vi "DataProcess_ChangeCatchName.vi"() -> ()   [LabVIEW 2016]
panel:
  in  "path 2":path
  out "Array 2":bool[](array[boolean])
  out "Array":string[](array[string])
  out "filenames":string[](array[string])
  in  "path":path
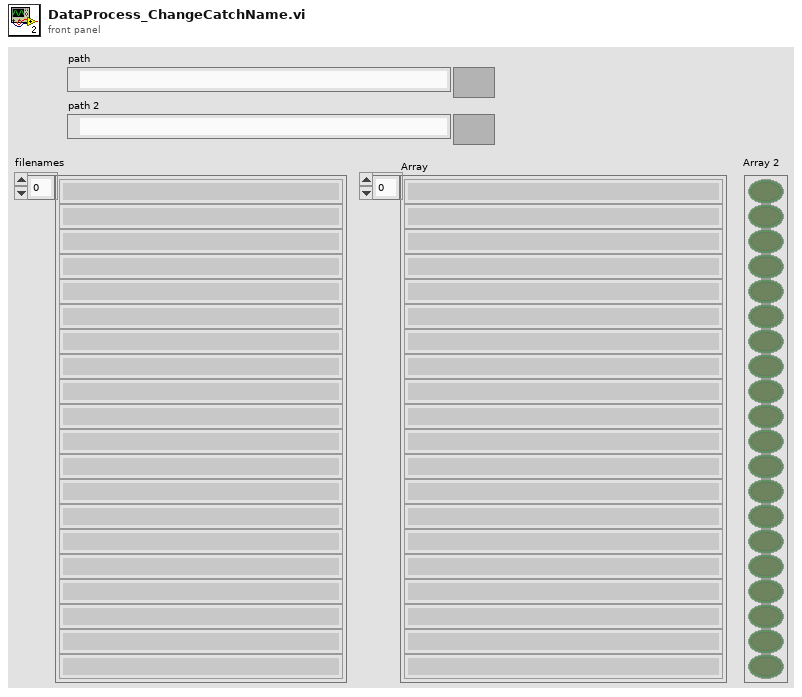
[diagram p1: front panel]
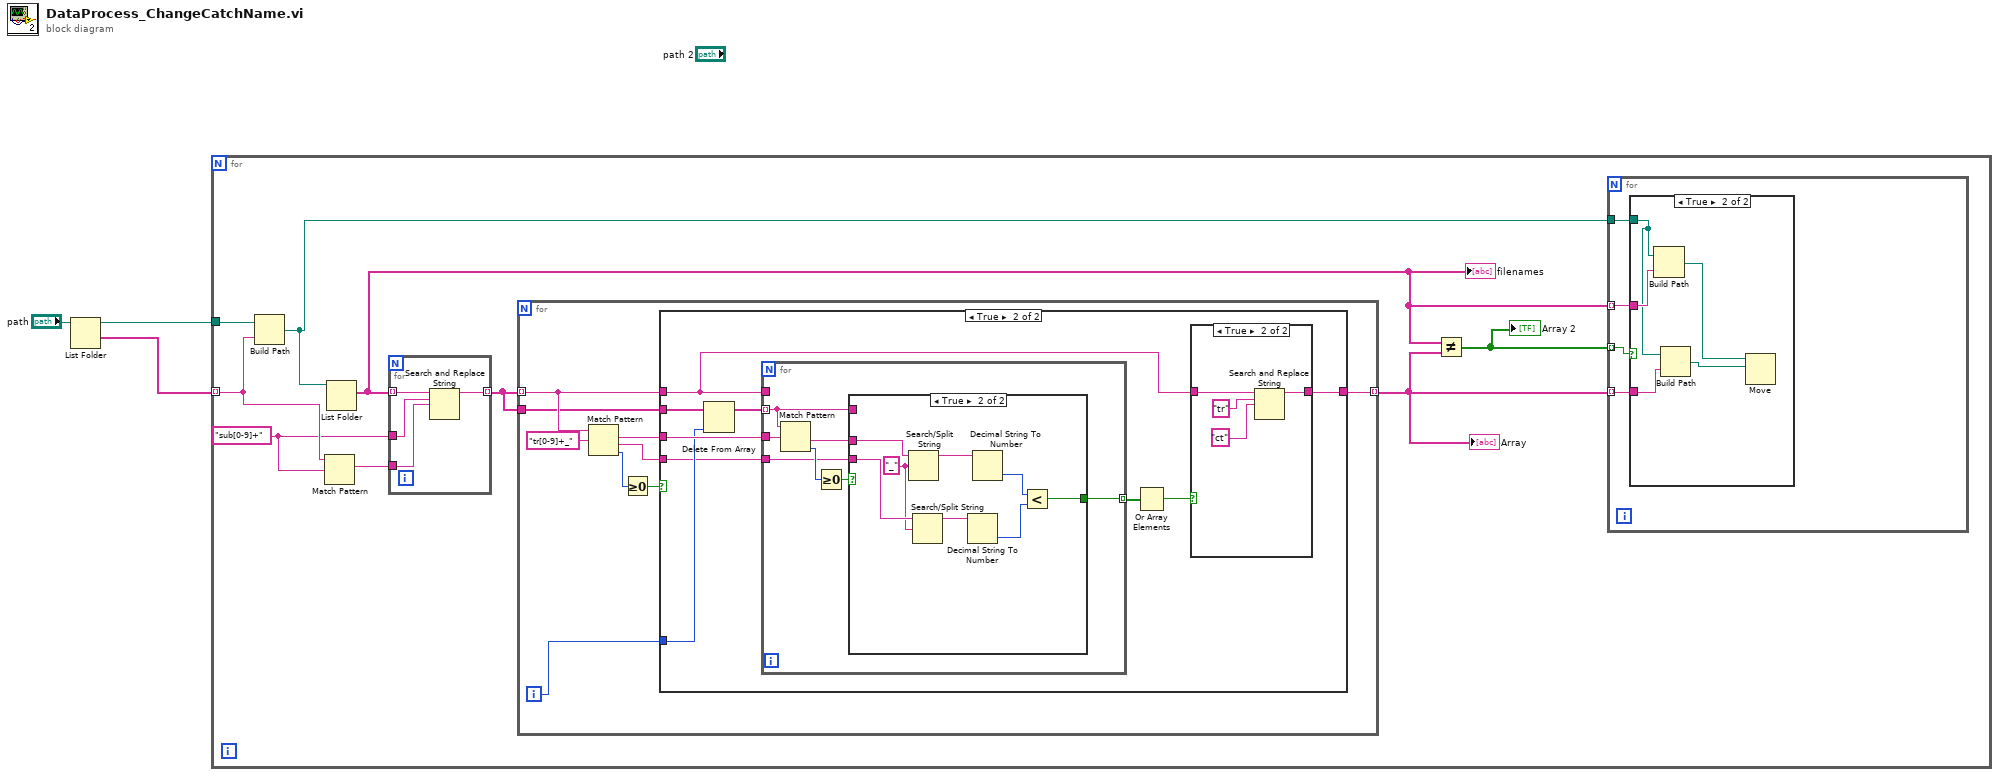
[diagram p0: block diagram]
diagram:
  n1 = List Folder(path="path") -> (path out=w1:path, folder names=w2:string[])  [unwired: 3 in, 2 out]
  n2 = for {
    tunnel: w2 -> [w11] mode=indexing
    tunnel: w1 -> [w12]
    w10 = "sub[0-9]+" ("search string")
    n3 = Build Path(base path=w12, name or relative path=w11) -> (appended path=w5:path)
    n4 = Match Pattern(string=w11, regular expression=w10) -> (match substring=w9:string)  [unwired: 1 in, 3 out]
    n5 = List Folder(path=w5) -> (filenames=w7:string[])  [unwired: 3 in, 3 out]
    "filenames" <- w7
    n6 = for {
      tunnel: w7 -> [w64] mode=indexing
      tunnel: w10 -> [w63]
      tunnel: w9 -> [w62]
      tunnel: [w61] -> w8 mode=indexing
      n7 = Search and Replace String(input string=w64, search string=w63, replace string=w62) -> (result string=w61:string)  [unwired: 5 in, 3 out]
    }
    n8 = for {
      tunnel: w8 -> [w25] mode=indexing
      tunnel: w8 -> [w24]
      tunnel: [w22] -> w6 mode=indexing
      i -> [w23]
      n9 = Match Pattern(string=w25, regular expression="tr[0-9]+_") -> (match substring=w27:string, after substring=w26:string, offset past match=w29:i32)  [unwired: 1 in, 1 out]
      n10 = Greater Or Equal To 0?(x=w29) -> (x >= 0?=w28:bool)
      n11 = case shown="True" w28 {
        tunnel: w27 -> [_ w40]
        tunnel: w26 -> [_ w36]
        tunnel: w25 -> [w31 w33]
        tunnel: w24 -> [_ w39]
        tunnel: w23 -> [_ w38]
        tunnel: [w31 w32] -> w22
        frame False {
        }
        frame True {
          n12 = Delete From Array(array=w39, index=w38) -> (array with subset deleted=w37:string[])  [unwired: 1 in, 1 out]
          n13 = for {
            tunnel: w37 -> [w49] mode=indexing
            tunnel: w40 -> [w52]
            tunnel: w36 -> [w47]
            tunnel: w33 -> [_]
            tunnel: [w46] -> w35 mode=indexing
            n14 = Match Pattern(string=w49, regular expression=w52) -> (after substring=w48:string, offset past match=w51:i32)  [unwired: 1 in, 2 out]
            n15 = Greater Or Equal To 0?(x=w51) -> (x >= 0?=w50:bool)
            n16 = case shown="True" w50 {
              tunnel: w49 -> [_ _]
              tunnel: w48 -> [_ w60]
              tunnel: w47 -> [_ w59]
              tunnel: [_ w53] -> w46
              frame False {
              }
              frame True {
                w58 = "_" ("search string/char (-)")
                n17 = Search/Split String(string=w60, search string/char (-)=w58) -> (substring before match=w57:string)  [unwired: 1 in, 2 out]
                n18 = Search/Split String(string=w59, search string/char (-)=w58) -> (substring before match=w56:string)  [unwired: 1 in, 2 out]
                n19 = Decimal String To Number(string=w56) -> (number=w54:i32)  [unwired: 2 in, 1 out]
                n20 = Decimal String To Number(string=w57) -> (number=w55:i32)  [unwired: 2 in, 1 out]
                n21 = Less?(x=w55, y=w54) -> (x < y?=w53:bool)
              }
            }
          }
          n22 = Or Array Elements(Boolean array=w35) -> (logical OR=w34:bool)
          n23 = case shown="True" w34 {
            tunnel: [w41 w43] -> w32
            tunnel: w33 -> [w41 w42]
            frame False {
            }
            frame True {
              n24 = Search and Replace String(input string=w42, search string="tr", replace string="ct" ("replace string (\"\")")) -> (result string=w43:string)  [unwired: 5 in, 3 out]
            }
          }
        }
      }
    }
    "Array" <- w6
    n25 = Not Equal?(x=w7, y=w6) -> (x != y?=w4:bool[])
    "Array 2" <- w4
    n26 = for {
      tunnel: w7 -> [w16] mode=indexing
      tunnel: w6 -> [w14] mode=indexing
      tunnel: w5 -> [w15]
      tunnel: w4 -> [w13] mode=indexing
      n27 = case shown="True" w13 {
        tunnel: w16 -> [_ w21]
        tunnel: w15 -> [_ w19]
        tunnel: w14 -> [_ w18]
        frame False {
        }
        frame True {
          n28 = Build Path(base path=w19, name or relative path=w21) -> (appended path=w20:path)
          n29 = Build Path(base path=w19, name or relative path=w18) -> (appended path=w17:path)
          n30 = Move(source path=w20, 10:w17) -> ()  [unwired: 3 in, 3 out]
        }
      }
    }
  }
